vi "CreateVINamesToReplace.vi"(7 "Foldername":string, 8 "NewVIName":string, 9 "BaseConstructorBase":path, 10 "TemplBaseConstructorBase":path) -> (1 "NewVIName":path, 3 "OldVIName":path)   [LabVIEW 2020, in "ClassWriterGOOP400.lvclass"]
uses:
  ClassWriterGOOP400.lvclass
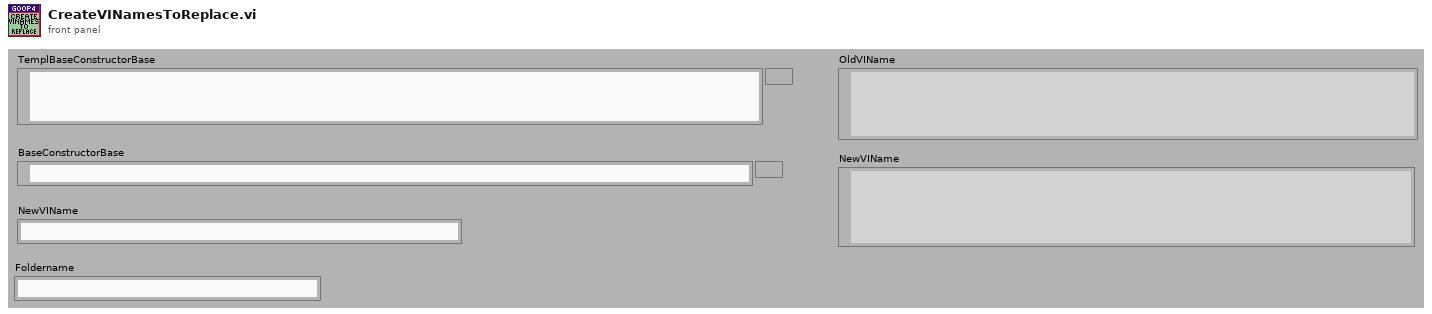
[diagram p1: front panel]
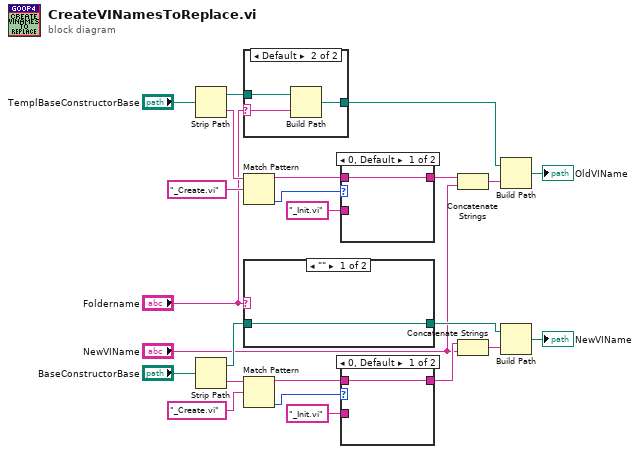
[diagram p0: block diagram]
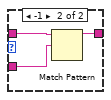
[diagram p2: hidden frame]
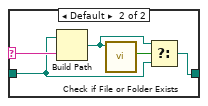
[diagram p3: hidden frame]
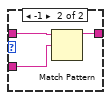
[diagram p4: hidden frame]
diagram:
  n1 = Strip Path(path="TemplBaseConstructorBase") -> (stripped path=w20:path, name=w18:string)
  n2 = Strip Path(path="BaseConstructorBase") -> (stripped path=w7:path, name=w9:string)
  n3 = case shown="Default" "Foldername" {
    selector: "Foldername" -> [_ w26]
    tunnel: [w25 w28] -> w22
    tunnel: w20 -> [w25 w27]
    frame "" {
    }
    frame Default {
      n4 = Build Path(base path=w27, name or relative path=w26) -> (appended path=w28:path)
    }
  }
  n5 = Match Pattern(string=w18, regular expression="_Create.vi") -> (before substring=w16:string, offset past match=w17:i32)  [unwired: 1 in, 2 out]
  n6 = case shown="\"\"" "Foldername" {
    selector: "Foldername" -> [_ w34]
    tunnel: [w29 w30] -> w5
    tunnel: w7 -> [w29 w32]
    frame "" {
    }
    frame Default {
      n7 = Build Path(base path=w32, name or relative path=w34) -> (appended path=w31:path)
      n8 = call <vilib>:"Check if File or Folder Exists.vi"("path"=w31) -> ("file or folder exists?"=w33:bool)  [unwired: 8 in, 2 out]
      n9 = Select(t=w31, s=w33, f=w32) -> (s? t:f=w30:path)
    }
  }
  n10 = Match Pattern(string=w9, regular expression="_Create.vi") -> (before substring=w11:string, offset past match=w10:i32)  [unwired: 1 in, 2 out]
  n11 = case shown="0, Default" w17 {
    tunnel: w16 -> [w35 w38]
    tunnel: "_Init.vi" -> [_ w37]
    tunnel: [w35 w36] -> w14
    frame 0, Default {
    }
    frame -1 {
      n12 = Match Pattern(string=w38, regular expression=w37) -> (before substring=w36:string)  [unwired: 1 in, 3 out]
    }
  }
  n13 = case shown="0, Default" w10 {
    tunnel: w11 -> [w39 w42]
    tunnel: "_Init.vi" -> [_ w41]
    tunnel: [w39 w40] -> w13
    frame 0, Default {
    }
    frame -1 {
      n14 = Match Pattern(string=w42, regular expression=w41) -> (before substring=w40:string)  [unwired: 1 in, 3 out]
    }
  }
  n15 = Concatenate Strings(w14, "NewVIName") -> (w21:string)
  n16 = Concatenate Strings(w13, "NewVIName") -> (w6:string)
  n17 = Build Path(base path=w22, name or relative path=w21) -> (appended path=→"OldVIName":path)
  n18 = Build Path(base path=w5, name or relative path=w6) -> (appended path=→"NewVIName":path)
